vi "Emerson 5700 Hot Water Calculation.vi"(7 "RTD Out (°F)":dbl, 8 "Error In":errorcluster, 11 "Emerson Flow Meter Data Output":T1) -> (0 "Error Out":errorcluster, 3 "Emerson Flow Meter Data Output 2":T1)   [LabVIEW 2016]
uses:
  Type Definitions/Emerson 5700 Data.ctl
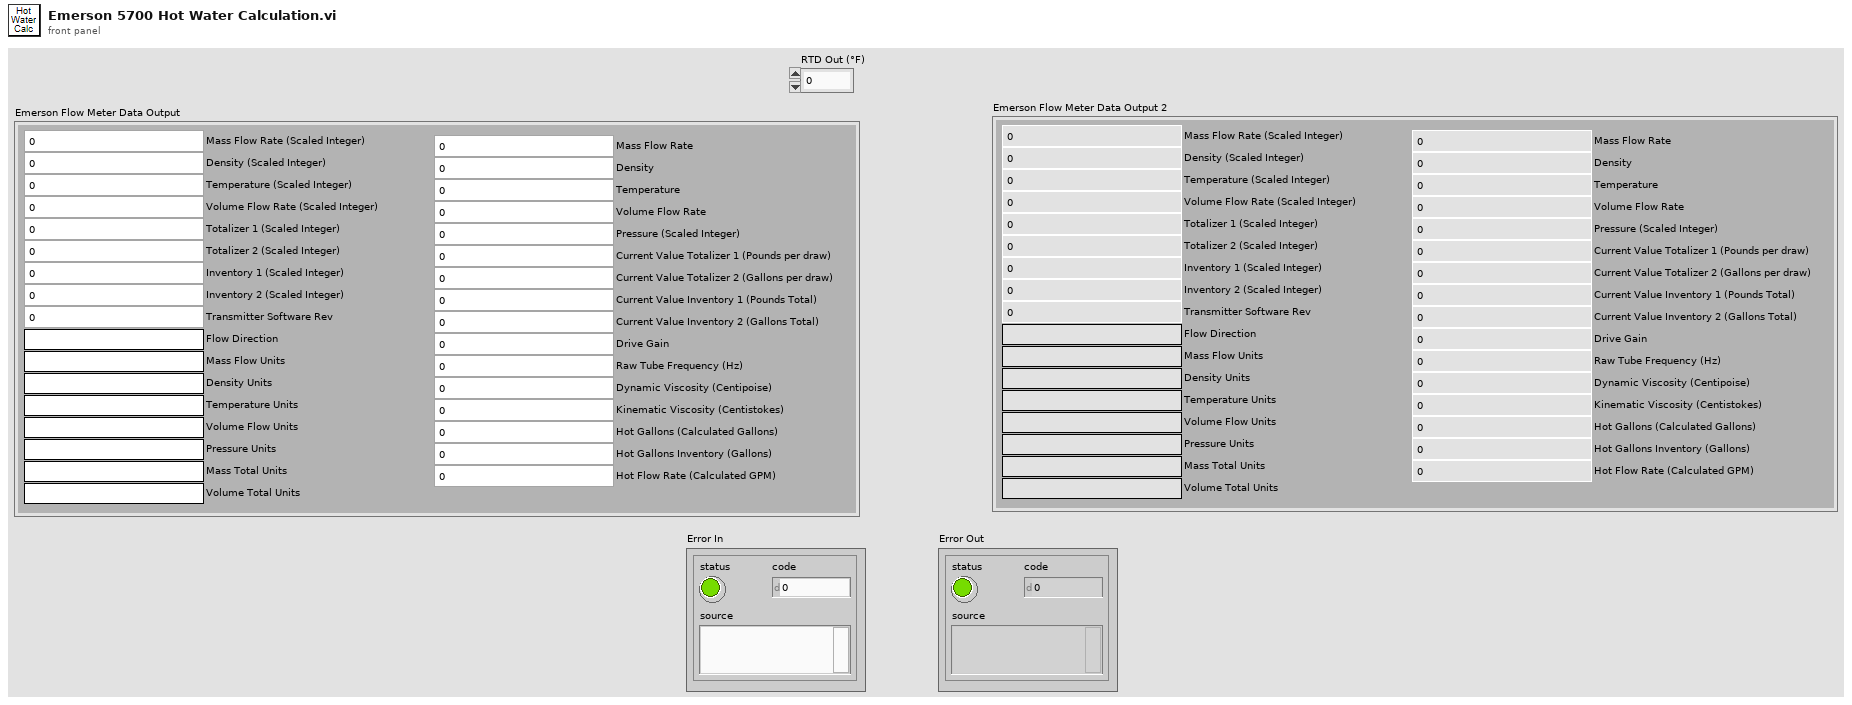
[diagram p1: front panel]
types:
  T1 = typedef "Emerson 5700 Data.ctl" = cluster{"Mass Flow Rate (Scaled Integer)":u16, "Density (Scaled Integer)":u16, "Temperature (Scaled Integer)":u16, "Volume Flow Rate (Scaled Integer)":u16, "Totalizer 1 (Scaled Integer)":u16, "Totalizer 2 (Scaled Integer)":u16, "Transmitter Software Rev":u16, "Flow Direction":string, "Mass Flow Units":string, "Density Units":string, "Temperature Units":string, "Volume Flow Units":string, "Pressure Units":string, "Mass Total Units":string, "Volume Total Units":string, "Inventory 1 (Scaled Integer)":u16, "Inventory 2 (Scaled Integer)":u16, "Mass Flow Rate":dbl, "Density":dbl, "Temperature":dbl, "Volume Flow Rate":dbl, "Pressure (Scaled Integer)":u16, "Current Value Totalizer 1 (Pounds per draw)":dbl, "Current Value Totalizer 2 (Gallons per draw)":dbl, "Current Value Inventory 1 (Pounds Total)":dbl, "Current Value Inventory 2 (Gallons Total)":dbl, "Drive Gain":dbl, "Raw Tube Frequency (Hz)":dbl, "Dynamic Viscosity (Centipoise)":dbl, "Kinematic Viscosity (Centistokes)":dbl, "Hot Gallons (Calculated Gallons)":dbl, "Hot Flow Rate (Calculated GPM)":dbl, "Hot Gallons Inventory (Gallons)":dbl}
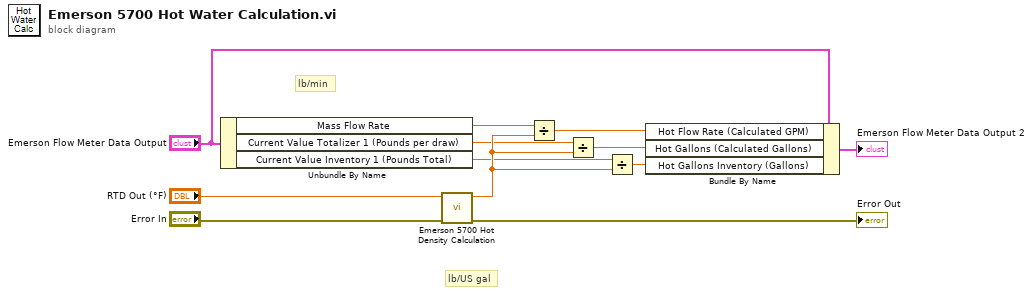
[diagram p0: block diagram]
diagram:
  # "lb/min"
  # "lb/US gal"
  n1 = Unbundle By Name("Emerson Flow Meter Data Output") -> ("Mass Flow Rate"=w10:dbl, "Current Value Totalizer 1 (Pounds per draw)"=w4:dbl, "Current Value Inventory 1 (Pounds Total)"=w3:dbl)
  n2 = call "Emerson 5700 Hot Density Calculation.vi"("Error In"="Error In", "RTD Out (°F)"="RTD Out (°F)") -> ("Error Out"=→"Error Out":errorcluster, "Density (lb/gal)"=w5:dbl)  [unwired: 8 in]
  n3 = Divide(x=w10, y=w5) -> (x/y=w8:dbl)
  n4 = Divide(x=w4, y=w5) -> (x/y=w2:dbl)
  n5 = Divide(x=w3, y=w5) -> (x/y=w1:dbl)
  n6 = Bundle By Name(cluster="Emerson Flow Meter Data Output", "Hot Flow Rate (Calculated GPM)"=w8, "Hot Gallons (Calculated Gallons)"=w2, "Hot Gallons Inventory (Gallons)"=w1) -> (→"Emerson Flow Meter Data Output 2":T1)
